vi "ITData_Rf.vi"(8 "error in (no error)":errorcluster, 11 "Data In":T1) -> (0 "error out":errorcluster, 3 "Data Out":T1)   [LabVIEW 2014]
uses:
  controls/Data.ctl
  <vilib>/Utility/file.llb/Write To Spreadsheet File (string).vi
panel:
  # "日期"
  # "機種名稱"
  # "機種代號"
  # "商品條碼"
  # "台"
  # "OK"
  # "NG"
  # "台"
  # "總計"
  # "台"
  # "日期"
  # "機種名稱"
  # "機種代號"
  # "商品條碼"
  # "台"
  # "OK"
  # "NG"
  # "台"
  # "總計"
  # "台"
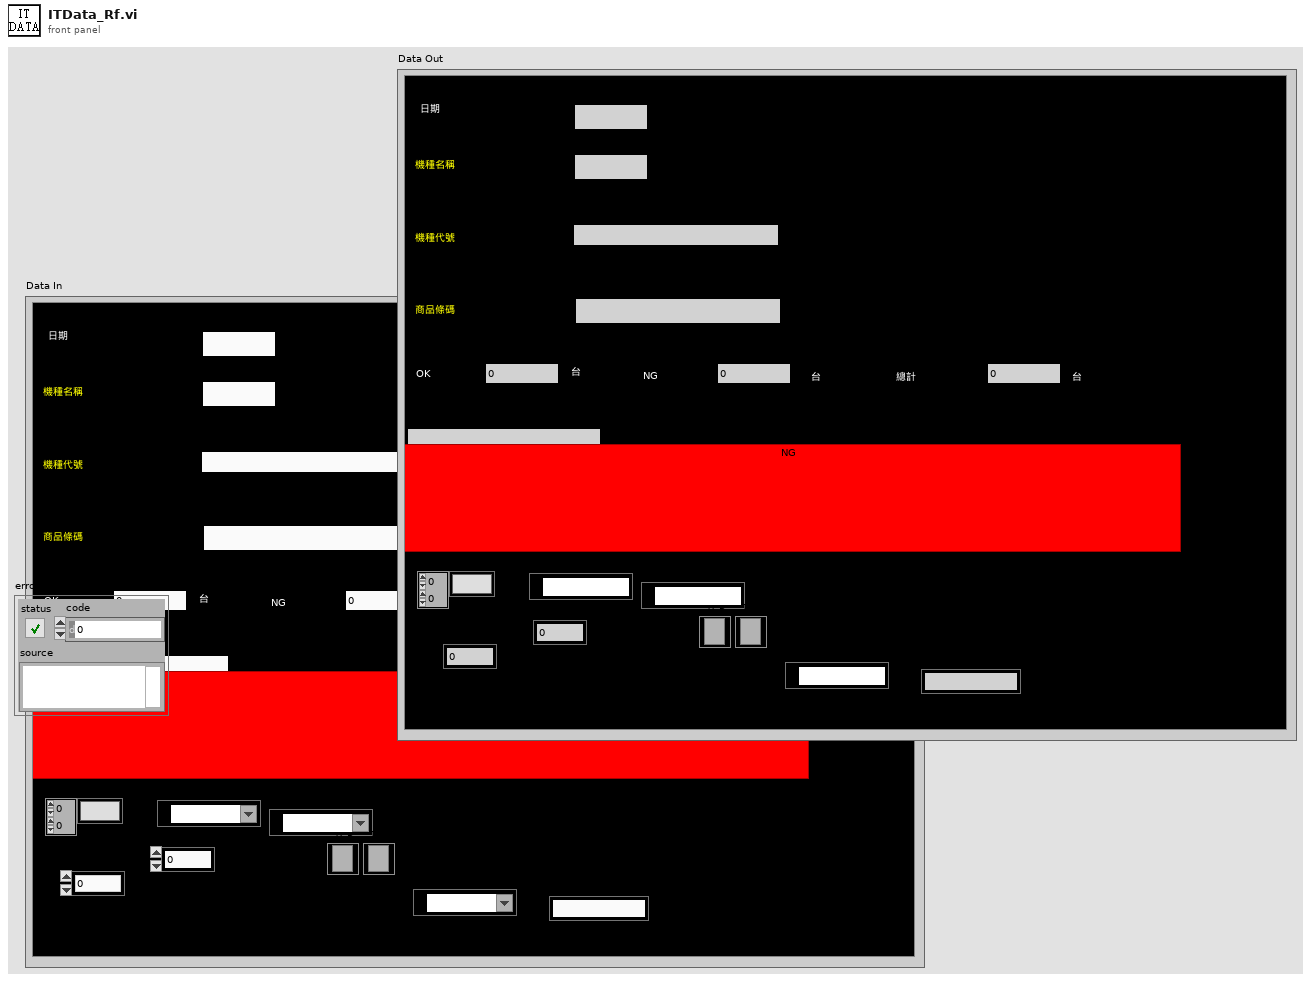
[diagram p1: front panel]
types:
  T1 = typedef "Data.ctl" = cluster{"Date":string, "BarCode1":string, "BarCode2":string, "BarCode3":string, "Message":string, "OK Count":u16, "NG Count":u16, "Total Count":u16, "ModelData":string[][], "OK&NG":bool, "COM1":refnum<visa-resource-name>, "COM2":refnum<visa-resource-name>, "IO":i32, "Time":u32, "TCP":refnum<k5>, "TCP 2":refnum<k5>, "COM3":refnum<visa-resource-name>, "CheckPars":string}
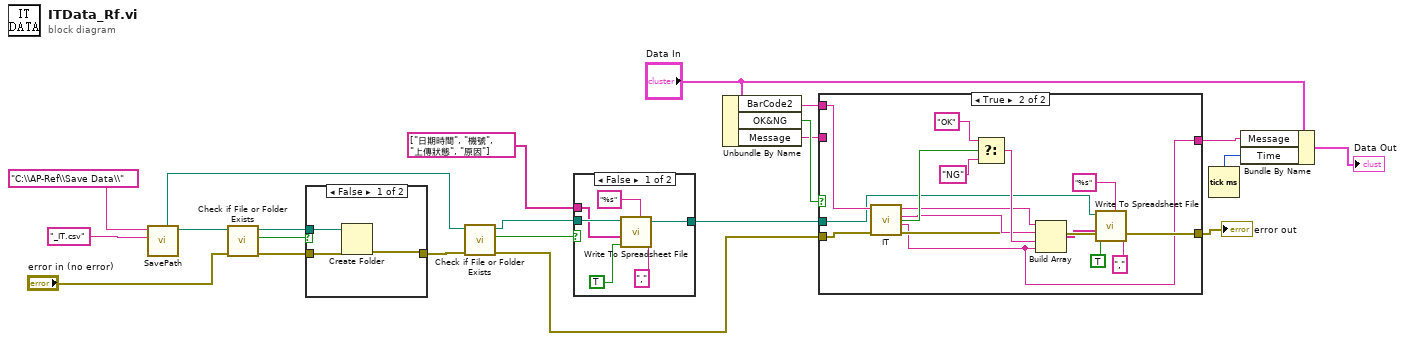
[diagram p0: block diagram]
diagram:
  n1 = call "SavePath.vi"("File Name"="_IT.csv", "Path In"="C:\\AP-Ref\\Save Data\\") -> ("Folder Path"=w22:path, "File Path"=w20:path)  [unwired: 8 in]
  n2 = call <vilib>:"Check if File or Folder Exists.vi"("error in (no error)"="error in (no error)", "path"=w22) -> ("error out"=w19:errorcluster, "file or folder exists?"=w21:bool, "dup path"=w17:path)  [unwired: 7 in]
  n3 = case shown="False" w21 {
    tunnel: w19 -> [w24 w26]
    tunnel: [w23 w26] -> w18
    tunnel: w17 -> [w25 _]
    frame False {
      n4 = Create Folder(path (use dialog)=w25, error in=w24) -> (error out=w23:errorcluster)  [unwired: 1 in, 2 out]
    }
    frame True {
    }
  }
  n5 = call <vilib>:"Check if File or Folder Exists.vi"("error in (no error)"=w18, "path"=w20) -> ("error out"=w7:errorcluster, "file or folder exists?"=w15:bool, "dup path"=w16:path)  [unwired: 7 in]
  n6 = case shown="False" w15 {
    tunnel: w16 -> [w32 w33]
    tunnel: [w30 w33] -> w9
    tunnel: string[] ["日期時間", "機號", "上傳狀態", "原因"] -> [w27 _]
    frame False {
      n7 = call-poly <vilib>:"Write To Spreadsheet File.vi"("delimiter (\\t)"="," ("delimiter (\\t)"), "format (%s)"="%s" ("format (%.3f)"), "append to file? (new file:F)"=TRUE, "1D data"=w27, "file path (dialog if empty)"=w32) -> ("new file path (Not A Path if cancelled)"=w30:path)  [unwired: 3 in]
    }
    frame True {
    }
  }
  n8 = Unbundle By Name("Data In") -> ("BarCode2"=w8:string, "OK&NG"=w10:bool, "Message"=w3:string)
  n9 = case shown="True" w10 {
    tunnel: w9 -> [_ w37]
    tunnel: w8 -> [_ w45]
    tunnel: w7 -> [w35 w44]
    tunnel: [w35 w39] -> w6
    tunnel: [w34 w36] -> w4
    tunnel: w3 -> [w34 _]
    frame False {
    }
    frame True {
      n10 = call "IT.vi"("error in (no error)"=w44, "機號"=w45) -> ("error out"=w39:errorcluster, "Msg"=w36:string, "BARCODE"=w40:string, "Date Time"=w41:string, "UP OK"=w43:bool)  [unwired: 4 in]
      n11 = Select(t="OK", s=w43, f="NG") -> (s? t:f=w42:string)
      n12 = Build Array(w41, w40, w42, w36) -> (w38:string[])
      n13 = call-poly <vilib>:"Write To Spreadsheet File.vi"("delimiter (\\t)"="," ("delimiter (\\t)"), "format (%s)"="%s", "append to file? (new file:F)"=TRUE, "1D data"=w38, "file path (dialog if empty)"=w37) -> ()  [unwired: 3 in, 1 out]
    }
  }
  "error out" <- w6
  n14 = Tick Count (ms)() -> (millisecond timer value=w2:u32)
  n15 = Bundle By Name(cluster="Data In", "Message"=w4, "Time"=w2) -> (→"Data Out":T1)
